vi "Data Set Application Operations.vi"(7 "Path (\"@SAVE\\mysavefile.dfl\")":string="@SAVE\\mysavefile.dfl", 8 "error in (no error)":errorcluster, 9 "Item Name (\"\")":string, 10 "Operation (Save)":i32(ring) items=["Save", "Recall"], 11 "VISA resource name":refnum<visa-resource-name>) -> (0 "error out":errorcluster, 3 "VISA resource name out":refnum<visa-resource-name>)   [LabVIEW 2020, in "Rohde&Schwarz CMXP Base.lvlib"]
doc: "This VI executes a partial recall or save, i.e. restores or saves the settings of a specific application from the specified file.\n\nAttributes:\nRSCMXPBASE_ATTR_DATA_SET_APPLICATION_SAVE\nRSCMXPBASE_ATTR_DATA_SET_APPLICATION_RESTORE\n\nRemote-control commands:\nMMEMory:STORe:ITEM\nMMEMory:LOAD:ITEM"
uses:
  <instrlib>/Rohde&Schwarz CMXP Base/Rohde&Schwarz CMXP Base.lvlib
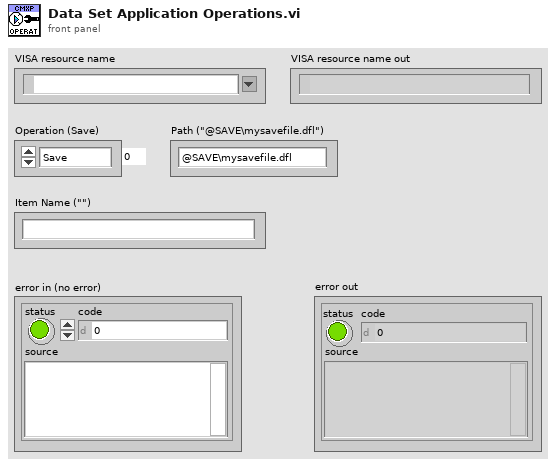
[diagram p1: front panel]
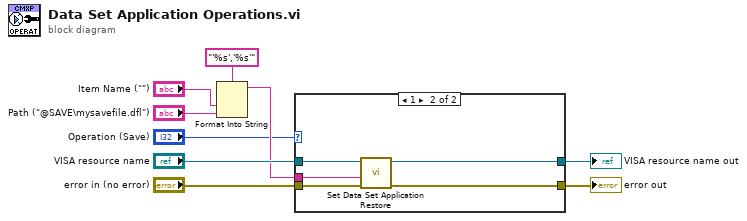
[diagram p0: block diagram]
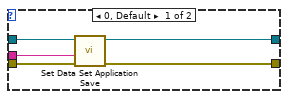
[diagram p2: hidden frame]
diagram:
  n1 = Format Into String(format string="'%s','%s'", "Item Name (\"\")", "Path (\"@SAVE\\mysavefile.dfl\")") -> (resulting string=w4:string)  [unwired: 2 in, 1 out]
  n2 = case shown="1" "Operation (Save)" {
    tunnel: "error in (no error)" -> [w14 w19]
    tunnel: "VISA resource name" -> [w13 w18]
    tunnel: [w12 w17] -> w7
    tunnel: [w11 w16] -> w6
    tunnel: w4 -> [w10 w15]
    frame 0, Default {
      n3 = call "Set Data Set Application Save"("error in (no error)"=w14, "Data Set Application Save ()"=w10, "instrument handle"=w13) -> ("error out"=w12:errorcluster, "instrument handle out"=w11:refnum<visa-resource-name>)  [unwired: 7 in]
    }
    frame 1 {
      n4 = call "Set Data Set Application Restore"("error in (no error)"=w19, "Data Set Application Restore ()"=w15, "instrument handle"=w18) -> ("error out"=w17:errorcluster, "instrument handle out"=w16:refnum<visa-resource-name>)  [unwired: 7 in]
    }
  }
  "error out" <- w7
  "VISA resource name out" <- w6
